vi "Read SSH.vi"(8 "Error In":errorcluster, 11 "Session In":refnum<class "Session.lvclass">) -> (0 "Erorr Out":errorcluster, 2 "SSH":refnum<class "SSH.lvclass">, 3 "Session Out":refnum<class "Session.lvclass">)   [LabVIEW 2021, in "Field_RnD_Services_LIBSSH2_Toolkit.lvlib" / "Session.lvclass"]
doc: "Gets the SSH context used to create this Session object and corresponding libssh2lv shared library Session struct."
uses:
  Session.lvclass
  SSH/SSH.lvclass
  Session.lvclass/Session.ctl
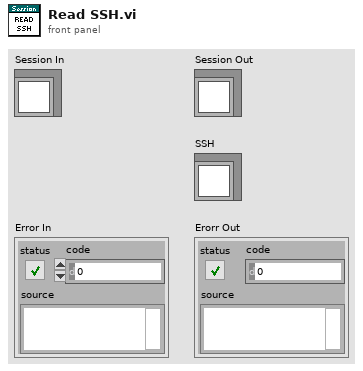
[diagram p1: front panel]
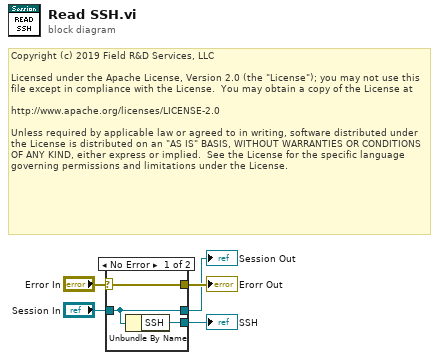
[diagram p0: block diagram]
diagram:
  # "Copyright (c) 2019 Field R&D Services, LLC\n\nLicensed under the Apache License, Version 2.0 (the \"License\"); you may not use this file except in compliance with the License.  You may obtain a copy of the License at\n\nhttp://www.apache.org/licenses/LICENSE-2.0\n\nUnless required by applicable law or agreed to in writing, software distributed under the License is distributed on an \"AS IS\" BASIS, WITHOUT WARRANTIES OR CONDITIONS OF ANY KIND, either express or implied.  See the License for the specific language governing permissions and limitations under the License."
  n1 = case shown="No Error" "Error In" {
    selector: "Error In" -> [w8 w9]
    tunnel: [w8 w9] -> w4
    tunnel: "Session In" -> [w7 w10]
    tunnel: [w7 w10] -> w2
    tunnel: [w6 _] -> w1
    frame No Error {
      n2 = Unbundle By Name(w7) -> ("SSH"=w6:refnum<class "SSH.lvclass">)
    }
    frame Error {
    }
  }
  "Erorr Out" <- w4
  "Session Out" <- w2
  "SSH" <- w1
